vi "GyroActions.vi"(10 "Update?":bool, 11 "Zero":bool) -> (0 "Yaw":dbl, 3 "YRPHfH":T1)   [LabVIEW 2018]
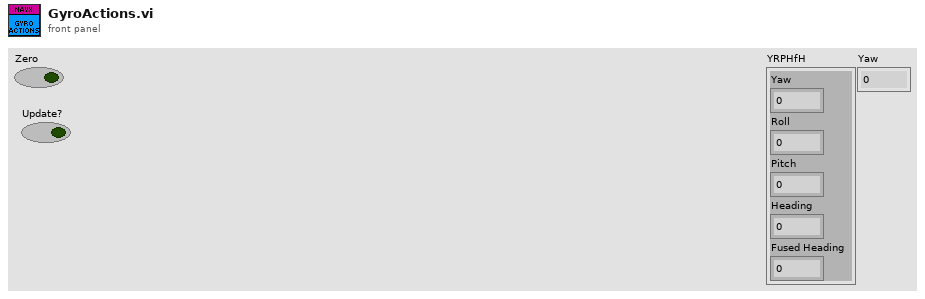
[diagram p1: front panel]
types:
  T1 = cluster{"Yaw":dbl, "Roll":dbl, "Pitch":dbl, "Heading":dbl, "Fused Heading":dbl}
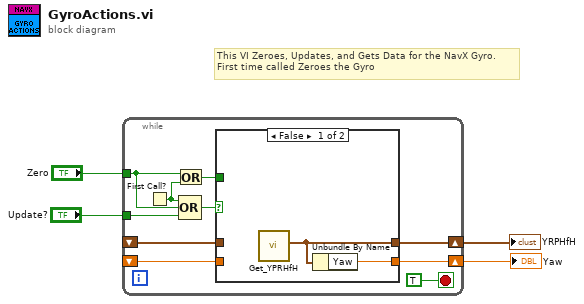
[diagram p0: block diagram]
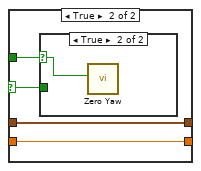
[diagram p2: hidden frame]
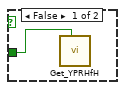
[diagram p3: hidden frame]
diagram:
  # "This VI Zeroes, Updates, and Gets Data for the NavX Gyro.\nFirst time called Zeroes the Gyro"
  n1 = while {
    tunnel: "Zero" -> [w11]
    tunnel: "Update?" -> [w10]
    shift-right: [w8] -> w2
    shift-left: _ -> [w6]
    shift-right: [w7] -> w1
    shift-left: _ -> [w5]
    stop <- TRUE stop-if-true
    n2 = First Call?() -> (First Call?: T/F=w12:bool)
    n3 = Or(x=w11, y=w12) -> (x .or. y?=w13:bool)
    n4 = Compound Arithmetic op=OR(w12, w11, w10) -> (w9:bool)
    n5 = case shown="False" w9 {
      selector: w9 -> [_ w19]
      tunnel: w13 -> [_ w20]
      tunnel: [w16 w18] -> w8
      tunnel: [w15 w17] -> w7
      tunnel: w6 -> [_ w18]
      tunnel: w5 -> [_ w17]
      frame False {
        n6 = call <vilib>:"Get_YPRHfH.vi"() -> ("YRPHfH"=w16:T1)  [unwired: 11 in]
        n7 = Unbundle By Name(w16) -> ("Yaw"=w15:dbl)
      }
      frame True {
        n8 = case shown="True" w20 {
          selector: w20 -> [_ w22]
          tunnel: w19 -> [w21 _]
          frame False {
            n9 = call <vilib>:"Get_YPRHfH.vi"("Update"=w21) -> ()  [unwired: 10 in, 1 out]
          }
          frame True {
            n10 = call <vilib>:"Zero Yaw.vi"("Zero"=w22) -> ()  [unwired: 11 in]
          }
        }
      }
    }
  }
  "YRPHfH" <- w2
  "Yaw" <- w1
